vi "Set Angle Unit.vi"(11 "angle units in":T1 items=["radian in, radian out", "radian in, degree out", "degree in, degree out", "degree in, radian out"]) -> (3 "angle units out":T1 items=["radian in, radian out", "radian in, degree out", "degree in, degree out", "degree in, radian out"])   [LabVIEW 2017, in "NI_AAL_Angle.lvlib"]
uses:
  <vilib>/Analysis/NI_AAL_Angle.lvlib
  <vilib>/Analysis/coordinate.llb/Angle Units.ctl
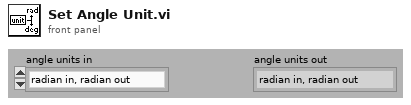
[diagram p1: front panel]
types:
  T1 = typedef "NI_AAL_Angle.lvlib/Angle Units.ctl" = i32
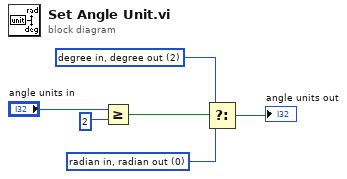
[diagram p0: block diagram]
diagram:
  w2 = T1 0 items=["radian in, radian out", "radian in, degree out", "degree in, degree out", "degree in, radian out"] ("angle units in 2")
  w1 = T1 2 items=["radian in, radian out", "radian in, degree out", "degree in, degree out", "degree in, radian out"] ("angle units in 2")
  n1 = Greater Or Equal?(x="angle units in", y=2) -> (x >= y?=w6:bool)
  n2 = Select(t=w1, s=w6, f=w2) -> (s? t:f=→"angle units out":T1)
